vi "tagDB Table Proble.vi"(11 "DB Ref":T2) -> (2 "Value String":string, 3 "Boolean":bool)   [LabVIEW 2014]
uses:
  TagDB/tagDB_Def.ctl
  TagDB/TagDB(dev).lvlib
panel:
  out "Valid?":bool
  out "Name":string
  out "DataItemFlag":i64
  out "DataChangeFlag":i64
  out "Array":T1(array[cluster])
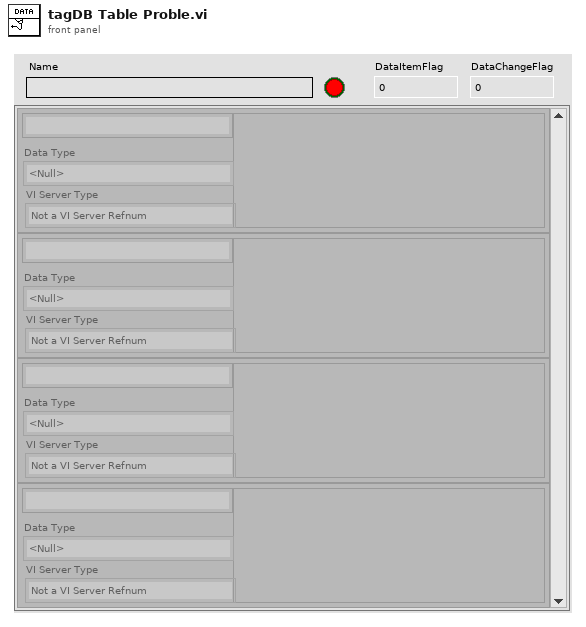
[diagram p1: front panel]
types:
  T1 = cluster{"Tag":string, "Data Type":enum8{"<Null>", "I8", "I16", "I32", "I64", "U8", "U16", "U32", "U64", "SGL", "DBL", "EXT", "CSG", "CDB", "CXT", "0x0F", "0x10", "0x11", "0x12", "0x13", "0x14", "Enum U8", "Enum U16", "Enum U32", "Enum U64", "SGL PQ", "DBL PQ", "EXT PQ", "CSG PQ", "CDB PQ", "CXT PQ", "0x1F", "0x20", "Boolean", "0x22", "0x23", "0x24", "0x25", "0x26", "0x27", "0x28", "0x29", "0x2A", "0x2B", "0x2C", "0x2D", "0x2E", "0x2F", "String", "0x31", "Path", "Pict", "0x34", "0x35", "0x36", "DAQ", "0x38", "0x39", "0x3A", "0x3B", "0x3C", "0x3D", "0x3E", "0x3F", "Array", "0x41", "0x42", "0x43", "0x44", "0x45", "0x46", "0x47", "0x48", "0x49", "0x4A", "0x4B", "0x4C", "0x4D", "0x4E", "0x4F", "Cluster", "0x51", "0x52", "Variant", "Waveform", "0x55", "0x56", "0x57", "0x58", "0x59", "0x5A", "0x5B", "0x5C", "0x5D", "0x5E", "0x5F", "0x60", "0x61", "0x62", "0x63", "0x64", "0x65", "0x66", "0x67", "0x68", "0x69", "0x6A", "0x6B", "0x6C", "0x6D", "0x6E", "0x6F", "Refnum"}, "VI Server Type":enum16{"Not a VI Server Refnum", "Control", "VI", "Application", "Splitter", "Pane"}, "Value":variant}[]
  T2 = typedef "TagDB(dev).lvlib/tagDB_Def.ctl" = refnum<k1>
  T3 = cluster{"Reference":refnum<vi>, "ClassName":string, "Value":variant}
  T4 = typedef "TagDB(dev).lvlib/_DEF-DATA.ctl" = cluster{"data hashmap":variant, "DataChangeFlag":i64, "ItemChangeFlag":i64, "name":string, "Tag Adding Lock?":bool}
  T5 = enum8{"<Null>", "I8", "I16", "I32", "I64", "U8", "U16", "U32", "U64", "SGL", "DBL", "EXT", "CSG", "CDB", "CXT", "0x0F", "0x10", "0x11", "0x12", "0x13", "0x14", "Enum U8", "Enum U16", "Enum U32", "Enum U64", "SGL PQ", "DBL PQ", "EXT PQ", "CSG PQ", "CDB PQ", "CXT PQ", "0x1F", "0x20", "Boolean", "0x22", "0x23", "0x24", "0x25", "0x26", "0x27", "0x28", "0x29", "0x2A", "0x2B", "0x2C", "0x2D", "0x2E", "0x2F", "String", "0x31", "Path", "Pict", "0x34", "0x35", "0x36", "DAQ", "0x38", "0x39", "0x3A", "0x3B", "0x3C", "0x3D", "0x3E", "0x3F", "Array", "0x41", "0x42", "0x43", "0x44", "0x45", "0x46", "0x47", "0x48", "0x49", "0x4A", "0x4B", "0x4C", "0x4D", "0x4E", "0x4F", "Cluster", "0x51", "0x52", "Variant", "Waveform", "0x55", "0x56", "0x57", "0x58", "0x59", "0x5A", "0x5B", "0x5C", "0x5D", "0x5E", "0x5F", "0x60", "0x61", "0x62", "0x63", "0x64", "0x65", "0x66", "0x67", "0x68", "0x69", "0x6A", "0x6B", "0x6C", "0x6D", "0x6E", "0x6F", "Refnum"}
  T6 = enum16{"Not a VI Server Refnum", "Control", "VI", "Application", "Splitter", "Pane"}
  T7 = cluster{string, "type":enum8{"<Null>", "I8", "I16", "I32", "I64", "U8", "U16", "U32", "U64", "SGL", "DBL", "EXT", "CSG", "CDB", "CXT", "0x0F", "0x10", "0x11", "0x12", "0x13", "0x14", "Enum U8", "Enum U16", "Enum U32", "Enum U64", "SGL PQ", "DBL PQ", "EXT PQ", "CSG PQ", "CDB PQ", "CXT PQ", "0x1F", "0x20", "Boolean", "0x22", "0x23", "0x24", "0x25", "0x26", "0x27", "0x28", "0x29", "0x2A", "0x2B", "0x2C", "0x2D", "0x2E", "0x2F", "String", "0x31", "Path", "Pict", "0x34", "0x35", "0x36", "DAQ", "0x38", "0x39", "0x3A", "0x3B", "0x3C", "0x3D", "0x3E", "0x3F", "Array", "0x41", "0x42", "0x43", "0x44", "0x45", "0x46", "0x47", "0x48", "0x49", "0x4A", "0x4B", "0x4C", "0x4D", "0x4E", "0x4F", "Cluster", "0x51", "0x52", "Variant", "Waveform", "0x55", "0x56", "0x57", "0x58", "0x59", "0x5A", "0x5B", "0x5C", "0x5D", "0x5E", "0x5F", "0x60", "0x61", "0x62", "0x63", "0x64", "0x65", "0x66", "0x67", "0x68", "0x69", "0x6A", "0x6B", "0x6C", "0x6D", "0x6E", "0x6F", "Refnum"}, "Enum":enum16{"Not a VI Server Refnum", "Control", "VI", "Application", "Splitter", "Pane"}, "Variant":variant}
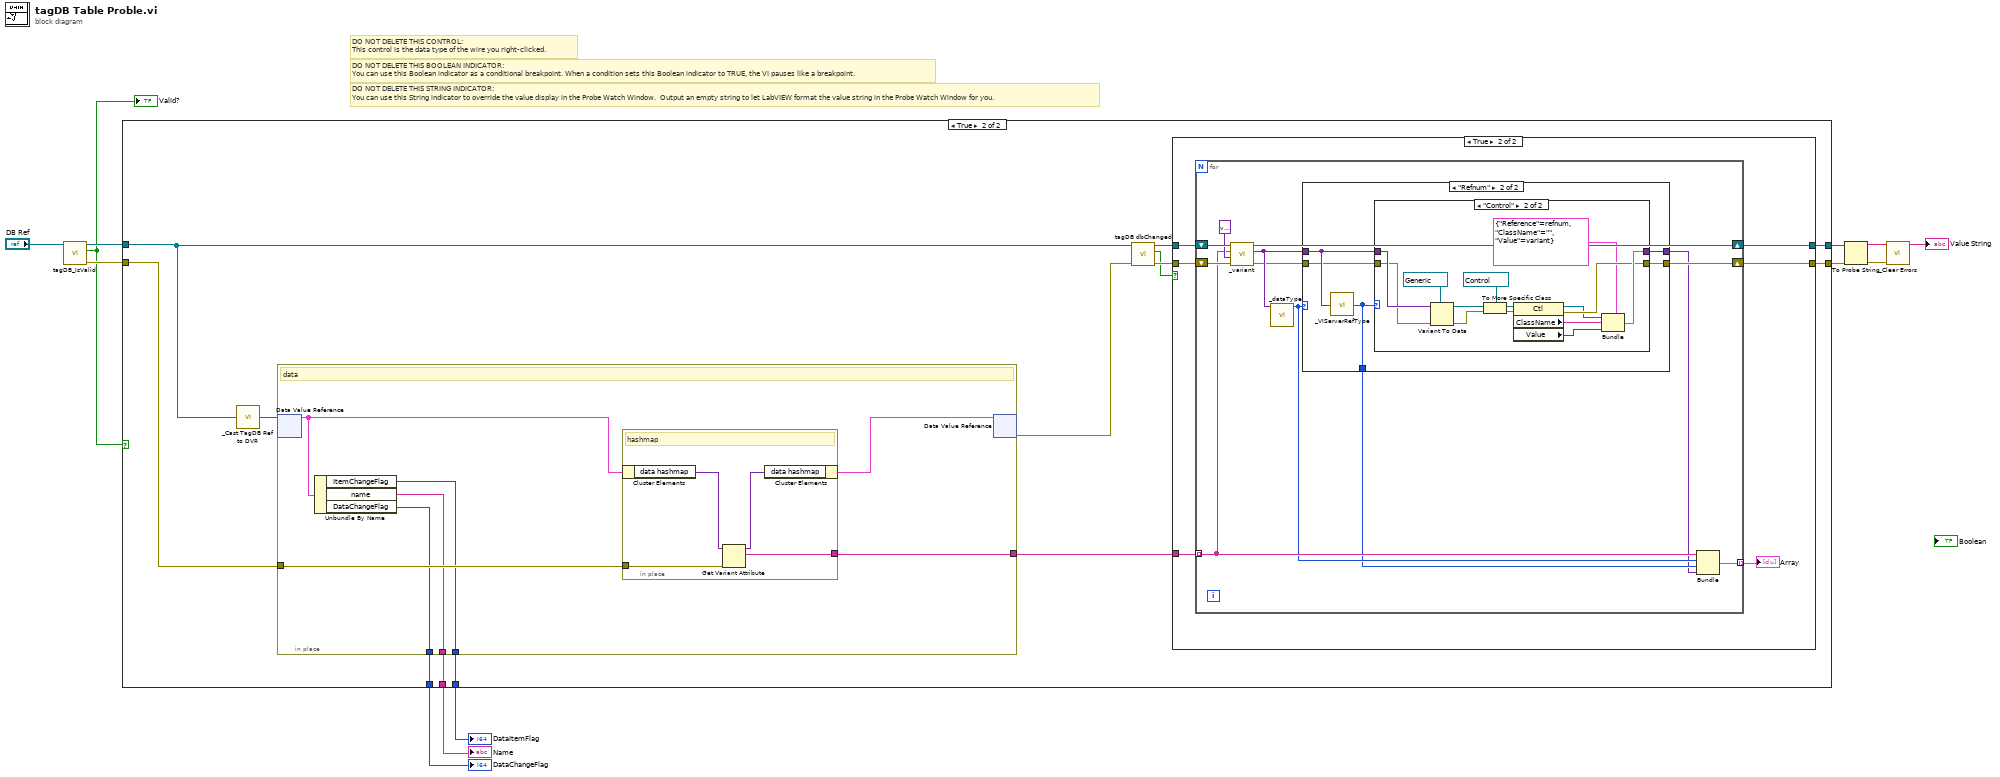
[diagram p0: block diagram]
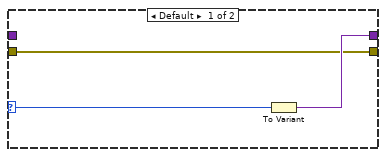
[diagram p5: hidden frame]
diagram:
  # "DO NOT DELETE THIS STRING INDICATOR: \nYou can use this String indicator to override the value display in the Probe Watch Window.  Output an empty string to let LabVIEW format the value string in the Probe Watch Window for you."
  # "DO NOT DELETE THIS BOOLEAN INDICATOR: \nYou can use this Boolean indicator as a conditional breakpoint. When a condition sets this Boolean indicator to TRUE, the VI pauses like a breakpoint."
  # "DO NOT DELETE THIS CONTROL: \nThis control is the data type of the wire you right-clicked."
  n1 = call "tagDB_IsValid.vi"("DB Ref in"="DB Ref") -> ("error out"=w8:errorcluster, "valid?"=w5:bool, "DB Ref out"=w9:T2)  [unwired: 8 in]
  "Valid?" <- w5
  n2 = case shown="True" w5 {
    tunnel: w9 -> [w13 w26]
    tunnel: w8 -> [w12 w25]
    tunnel: [w13 w23] -> w7
    tunnel: [w12 w22] -> w6
    tunnel: [_ w16] -> w3
    tunnel: [_ w15] -> w2
    tunnel: [_ w14] -> w1
    frame False {
    }
    frame True {
      n3 = call "_Cast TagDB Ref to DVR.vi"("TagDB"=w26) -> ("DVR"=w24:refnum<data-value>)  [unwired: 4 in]
      n4 = in-place {
        in-place-border: [w76] -> w21
        in-place-border: w25 -> [w74]
        in-place-border: [w73] -> w16
        in-place-border: [w72] -> w15
        in-place-border: [w71] -> w14
        # "data"
        n5 = in-place-dvr #1(w24) -> (w75:T4)  [unwired: 1 out]
        n6 = Unbundle By Name(w75) -> ("ItemChangeFlag"=w73:i64, "name"=w72:string, "DataChangeFlag"=w71:i64)
        n7 = in-place {
          in-place-border: [w79] -> w76
          in-place-border: w74 -> [w78]
          # "hashmap"
          n8 = in-place-cluster #2(w75) -> ("data hashmap"=w81:variant)
          n9 = Get Variant Attribute(Variant=w81, error in=w78) -> (duplicate Variant=w80:variant, names=w79:string[])  [unwired: 2 in, 2 out]
          n10 = in-place-cluster #2("data hashmap"=w80) -> (w77:T4)
        }
        n11 = in-place-dvr #1(w77) -> (w19:errorcluster)  [unwired: 1 out]
      }
      n12 = call "tagDB dbChanged.vi"("error in (no error)"=w19, "DB Ref"=w26) -> ("error in (no error) (dup)"=w18:errorcluster, "changed?"=w17:bool, "DB Ref (dup)"=w20:T2)  [unwired: 7 in]
      n13 = case shown="True" w17 {
        tunnel: [w28 w34] -> w23
        tunnel: [w27 w33] -> w22
        tunnel: w21 -> [_ w32]
        tunnel: w20 -> [w28 w31]
        tunnel: w18 -> [w27 w30]
        frame False {
        }
        frame True {
          n14 = for {
            tunnel: w32 -> [w39] mode=indexing
            shift-right: [w45] -> w34
            shift-left: w31 -> [w46]
            shift-right: [w44] -> w33
            shift-left: w30 -> [w43]
            tunnel: [w35] -> w29 mode=indexing
            n15 = call "_variant.vi"("error in (no error)"=w43, "default value (empty variant)"=variant, "name"=w39, "DB Ref"=w46) -> ("error out"=w40:errorcluster, "value"=w41:variant, "DB Ref (dup)"=w45:T2)  [unwired: 5 in]
            n16 = call "_dataType.vi"("Type"=w41) -> ("type"=w38:T5)  [unwired: 10 in]
            n17 = case shown="\"Refnum\"" w38 {
              tunnel: [w48 w53] -> w36
              tunnel: w41 -> [w48 w52]
              tunnel: w40 -> [w47 w51]
              tunnel: [w47 w50] -> w44
              tunnel: [_ w49] -> w37
              frame Default {
              }
              frame "Refnum" {
                n18 = call "_VIServerRefType.vi"("Data"=w52) -> ("Enum"=w49:T6)  [unwired: 4 in]
                n19 = case shown="\"Control\"" w49 {
                  selector: w49 -> [w56 _]
                  tunnel: [w55 w61] -> w53
                  tunnel: w52 -> [_ w70]
                  tunnel: w51 -> [w54 w60]
                  tunnel: [w54 w59] -> w50
                  frame Default {
                    n20 = To Variant(anything=w56) -> (Variant=w55:variant)
                  }
                  frame "Control" {
                    n21 = Variant To Data(error in=w60, type=refnum<vi> refnum ("value"), Variant=w70) -> (data=w68:refnum<vi>, error out=w67:errorcluster)
                    n22 = To More Specific Class(target class=refnum<vi> refnum ("value"), reference=w68, error in=w67) -> (specific class reference=w65:refnum<vi>, error out=w64:errorcluster)
                    n23 = property class="Ctl"(reference=w65, error in=w64) -> (reference out=w58:refnum<vi>, error out=w59:errorcluster, "ClassName"=w63:string, "Value"=w62:variant)
                    n24 = Bundle(cluster=T3 {"Reference"=refnum, "ClassName"="", "Value"=variant}, "Reference"=w58, "ClassName"=w63, "Value"=w62) -> (w61:T3)
                  }
                }
              }
            }
            n25 = Bundle(w39, "type"=w38, "Enum"=w37, "Variant"=w36) -> (w35:T7)  [unwired: 1 in]
          }
          "Array" <- w29
        }
      }
    }
  }
  "DataChangeFlag" <- w1
  "DataItemFlag" <- w3
  "Name" <- w2
  n26 = To Probe String(4:w6, 7:w7) -> (0:w4:errorcluster, 3:→"Value String":string)  [unwired: 1 in]
  n27 = call "_Clear Errors.vi"("error in (no error)"=w4) -> ()  [unwired: 5 in, 2 out]
